vi "STARTFIX2.vi"() -> ()   [LabVIEW 2024]
uses:
  <vilib>/Utility/file.llb/Read Delimited Spreadsheet (DBL).vi
panel:
  in  "Flow Rate Lower Limit 2":dbl
  in  "Flow Rate Upper Limit 2":dbl
  in  "Desired Flow Rate 3":dbl format="%_2f"
  in  "Initial RPM  3":dbl format="%_4f"
  in  "stop 2":bool
  out "Boolean":bool
  out "Waveform Chart 3":dbl[](graph)
  out "Waveform Chart 2":dbl[](graph)
  out "Flow Rate":dbl[](graph)
  in  "Color Box":u32(colorbox)
  # "Blood Flow Rate"
  # "Flow Rate (mL/min)"
  # "Initial LVAD Speed (RPM)"
  # "Desired Flow Rate (mL/min)"
  # "LVAD Speed"
  # "Upper Flow Rate Limit (mL/min)"
  # "Speed (RPM)"
  # "Lower Flow Rate Limit (mL/min)"
  # "Optimal Flow State"
  # "Right Heart Waveform"
  # "Amplitude"
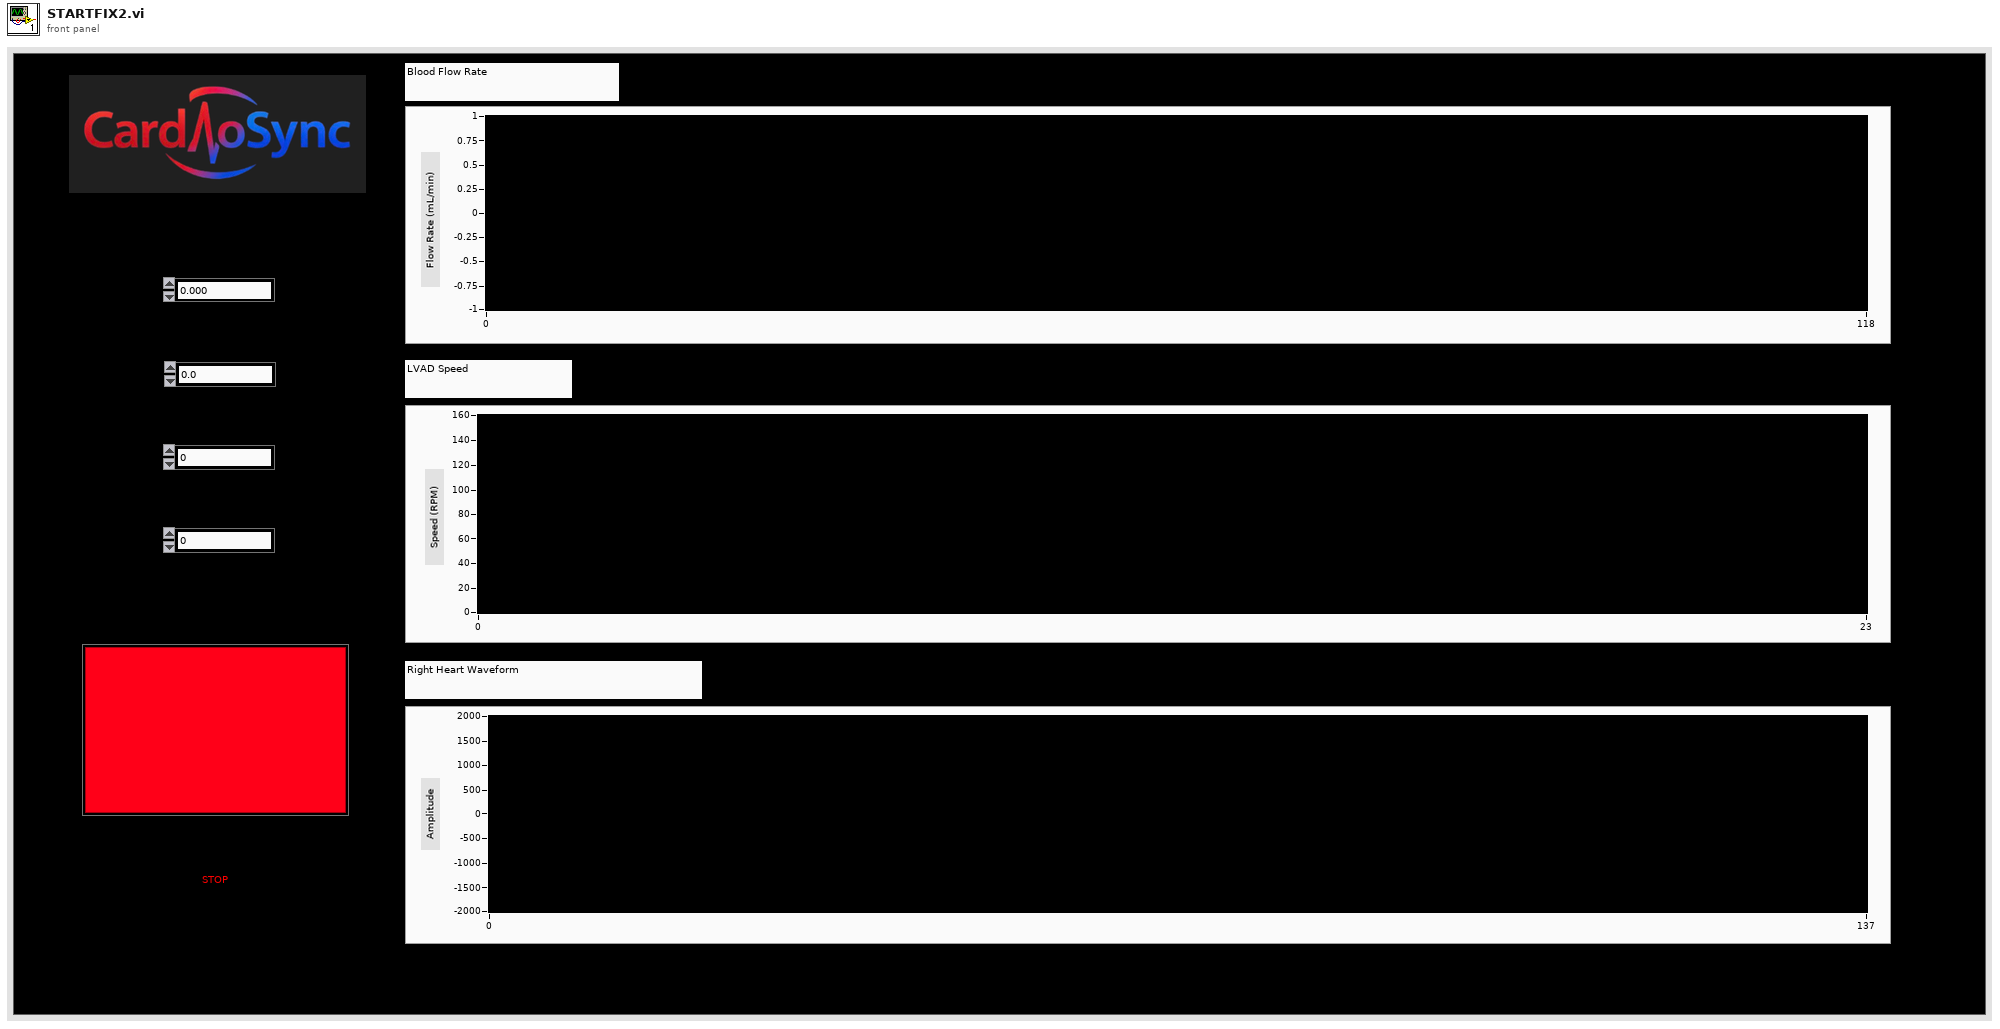
[diagram p1: front panel]
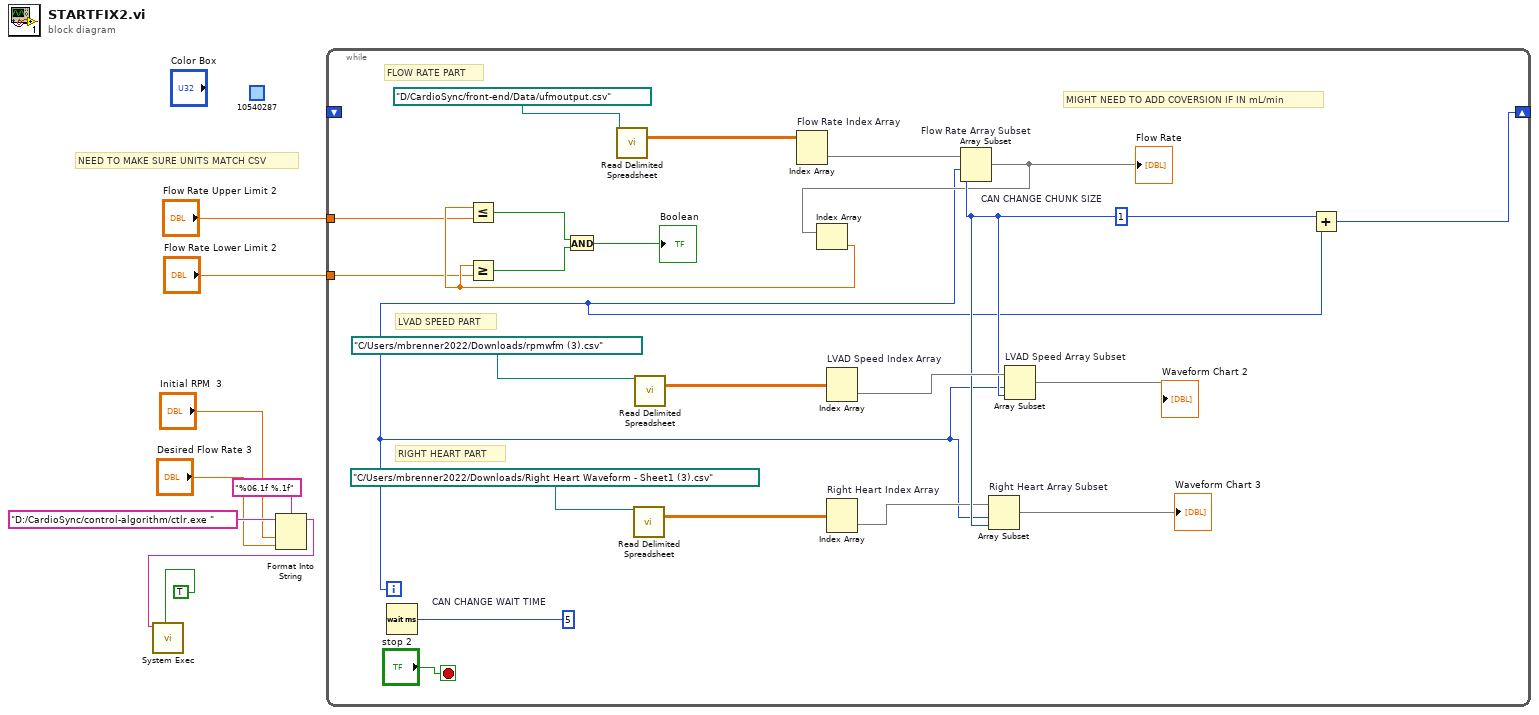
[diagram p0: block diagram]
diagram:
  (unwired) u32 10540287 ("Color Box 2")
  # "NEED TO MAKE SURE UNITS MATCH CSV"
  n1 = Format Into String(format string="%06.1f %.1f", initial string="D:/CardioSync/control-algorithm/ctlr.exe ", "Initial RPM  3", "Desired Flow Rate 3") -> (resulting string=w2:string)  [unwired: 1 in, 1 out]
  n2 = call <vilib>:"System Exec.vi"("wait until completion? (T)"=TRUE, "command line"=w2) -> ()  [unwired: 6 in, 4 out]
  n3 = while {
    shift-right: [w27] -> _
    shift-left: _ -> [_]
    tunnel: "Flow Rate Upper Limit 2" -> [w11]
    tunnel: "Flow Rate Lower Limit 2" -> [w10]
    i -> [w9]
    stop <- "stop 2" stop-if-true
    w28 = u32 5  # CAN CHANGE WAIT TIME
    w22 = 1  # CAN CHANGE CHUNK SIZE
    # "MIGHT NEED TO ADD COVERSION IF IN mL/min"
    # "RIGHT HEART PART"
    # "LVAD SPEED PART"
    # "FLOW RATE PART"
    n4 = Wait (ms)(milliseconds to wait=w28) -> ()  [unwired: 1 out]
    n5 = call-poly <vilib>:"Read Delimited Spreadsheet.vi"("file path (dialog if empty)"=path "D:/CardioSync/front-end/Data/ufmoutput.csv") -> ("all rows"=w30:dbl[][])  [unwired: 9 in, 5 out]
    n6 = call-poly <vilib>:"Read Delimited Spreadsheet.vi"("file path (dialog if empty)"=path "C:/Users/mbrenner2022/Downloads/Right Heart Waveform - Sheet1 (3).csv") -> ("all rows"=w23:dbl[][])  [unwired: 9 in, 5 out]
    n7 = call-poly <vilib>:"Read Delimited Spreadsheet.vi"("file path (dialog if empty)"=path "C:/Users/mbrenner2022/Downloads/rpmwfm (3).csv") -> ("all rows"=w25:dbl[][])  [unwired: 9 in, 5 out]
    n8 = Index Array "Flow Rate Index Array"(array=w30) -> (element=w29:dbl[])  [unwired: 2 in]
    n9 = Index Array "LVAD Speed Index Array"(array=w25) -> (element=w24:dbl[])  [unwired: 2 in]
    n10 = Index Array "Right Heart Index Array"(array=w23) -> (element=w18:dbl[])  [unwired: 2 in]
    n11 = Array Subset "Flow Rate Array Subset"(array=w29, index=w9, length=w22) -> (w14:dbl[])
    "Flow Rate" <- w14
    n12 = Index Array(array=w14) -> (element=w13:dbl)  [unwired: 1 in]
    n13 = Less Or Equal?(x=w13, y=w11) -> (x <= y?=w17:bool)
    n14 = Greater Or Equal?(x=w13, y=w10) -> (x >= y?=w16:bool)
    n15 = And(x=w17, y=w16) -> (x .and. y?=→"Boolean":bool)
    n16 = Array Subset "Right Heart Array Subset"(array=w18, index=w9, length=w22) -> (→"Waveform Chart 3":dbl[])
    n17 = Array Subset "LVAD Speed Array Subset"(array=w24, index=w9, length=w22) -> (→"Waveform Chart 2":dbl[])
    n18 = Add(x=w22, y=w9) -> (x+y=w27:i32)
  }
